vi "Pix_to_angle_velocity.vi"(11 "Pixel distance from cntr":dbl=7.5) -> (2 "V (km/s)":dbl=7.5, 3 "Angle out int (deg)":dbl=7.5, 5 "Angle in ext (deg)":dbl=7.5)   [LabVIEW 2012]
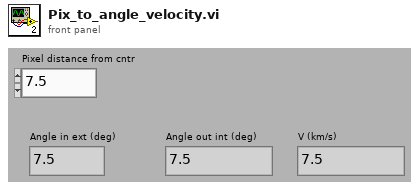
[diagram p1: front panel]
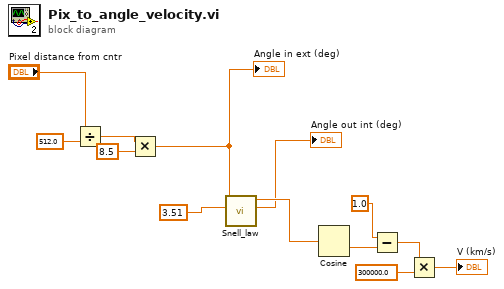
[diagram p0: block diagram]
diagram:
  n1 = Divide(x="Pixel distance from cntr", y=512.0) -> (x/y=w11:dbl)
  n2 = Multiply(x=w11, y=8.5) -> (x*y=w8:dbl)
  "Angle in ext (deg)" <- w8
  n3 = call "Snell_law.vi"("Refr index"=3.51, "Angle in ext (deg)"=w8) -> ("Angle out int (deg)"=→"Angle out int (deg)":dbl, "Angle out int (rad)"=w3:dbl)  [unwired: 8 in]
  n4 = Cosine(x=w3) -> (cos(x)=w7:dbl)
  n5 = Subtract(x=1.0, y=w7) -> (x-y=w5:dbl)
  n6 = Multiply(x=w5, y=300000.0) -> (x*y=→"V (km/s)":dbl)
